vi "get_size.vi"(8 "error in (no error)":errorcluster, 11 "PointCollection in":refnum<class "PointCollection.lvclass">) -> (0 "error out":errorcluster, 2 "number of points":i32, 3 "PointCollection out":refnum<class "PointCollection.lvclass">)   [LabVIEW 2010, in "PointCollection.lvclass"]
uses:
  PointCollection.lvclass
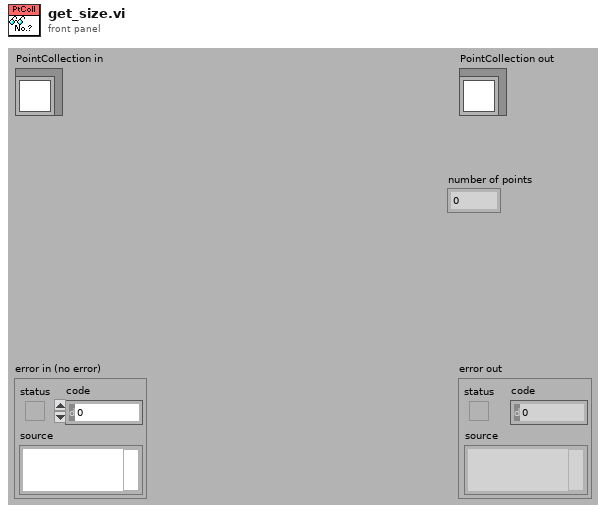
[diagram p1: front panel]
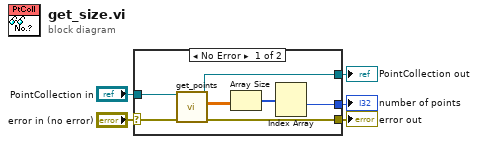
[diagram p0: block diagram]
diagram:
  n1 = case shown="No Error" "error in (no error)" {
    selector: "error in (no error)" -> [w11 w14]
    tunnel: [w10 w14] -> w4
    tunnel: [w7 w13] -> w2
    tunnel: "PointCollection in" -> [w8 w13]
    tunnel: [w6 _] -> w1
    frame No Error {
      n2 = call-dynamic "get_points.vi"("error in (no error)"=w11, "PointCollection in"=w8) -> ("error out"=w10:errorcluster, "points"=w12:dbl[][], "PointCollection out"=w7:refnum<class "PointCollection.lvclass">)  [unwired: 7 in]
      n3 = Array Size(array=w12) -> (size(s)=w9:i32[])
      n4 = Index Array(array=w9) -> (element #1=w6:i32)  [unwired: 2 in, 1 out]
    }
    frame Error {
    }
  }
  "error out" <- w4
  "PointCollection out" <- w2
  "number of points" <- w1
